vi "U3 Quadrature.vi"(8 "error in":errorcluster) -> (0 "error out":errorcluster)   [LabVIEW 2021]
panel:
  in  "Case Constant\n(See Context Help)":bool=TRUE
  in  "Stop":bool
  in  "Reset Count":bool
  out "Quadrature Count":i32
  in  "FirstFound":bool=TRUE
  in  "Address":string="1"
  out "Error Message":string
  # "Demonstrates 1 quadrature input, which uses two timer channels for phases A and B (FIO0 and FIO1 in this case).\nIf you don't have a quadrature signal source handy, you can connect wires to GND, and tap these wires on FIO0\nand FIO1 to simulate quadrature."
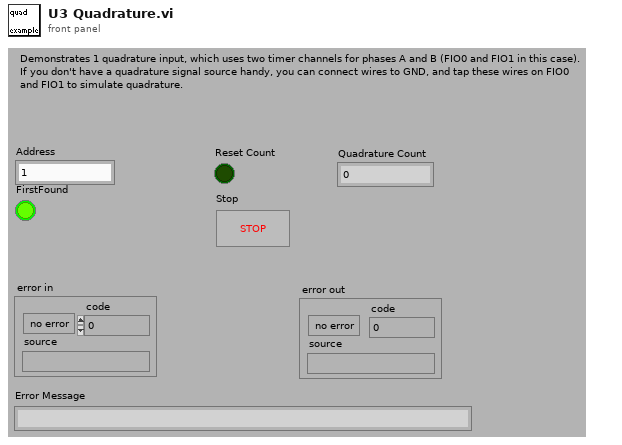
[diagram p1: front panel]
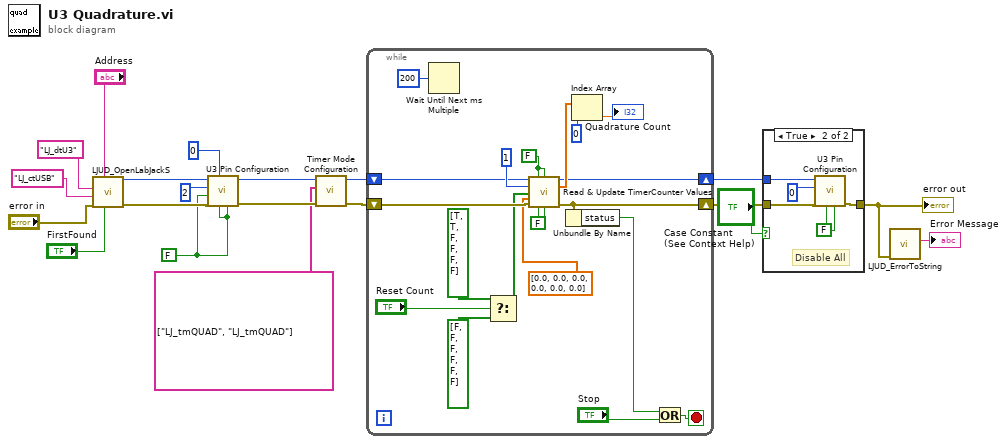
[diagram p0: block diagram]
diagram:
  w5 = FALSE ("Enable Counter0")
  n1 = call "LJUD_OpenLabJackS.vi"("FirstFound"="FirstFound", "Address"="Address", "error in"="error in", "ConnectionType"="LJ_ctUSB", "DeviceType"="LJ_dtU3") -> ("error out"=w8:errorcluster, "Handle"=w7:i32)  [unwired: 4 in, 1 out]
  n2 = call "U3 Pin Configuration.vi"("Enable Counter1"=w5, "Enable Counter0"=w5, "FIO/EIO Analog Enable"=0, "error in"=w8, "Enable DAC1"=w5, "Number of Timers Enabled"=2 ("# Timers Enabled"), "Handle In"=w7) -> ("error out"=w9:errorcluster, "Handle Out"=w6:i32)  [unwired: 3 in]
  n3 = call "Timer Mode Configuration.vi"("error in"=w9, "TimerModes"=string[] ["LJ_tmQUAD", "LJ_tmQUAD"], "Handle In"=w6) -> ("error out"=w14:errorcluster, "Handle Out"=w13:i32)  [unwired: 7 in]
  n4 = while {
    shift-right: [w32] -> w11
    shift-left: w13 -> [w34]
    shift-right: [w27] -> w12
    shift-left: w14 -> [w33]
    stop <- w26 stop-if-true
    w21 = FALSE ("Reset Counter0")
    w39 = FALSE ("Reset Counter0")
    n5 = Wait Until Next ms Multiple(millisecond multiple=u32 200) -> ()  [unwired: 1 out]
    n6 = Select(t=bool[] [TRUE, TRUE, FALSE, FALSE, FALSE, FALSE] ("UpdateReset Timers"), s="Reset Count", f=bool[] [FALSE, FALSE, FALSE, FALSE, FALSE, FALSE] ("UpdateReset Timers")) -> (s? t:f=w28:bool[])
    n7 = call "Read & Update TimerCounter Values.vi"("Handle In"=w34, "Reset Counter0"=w39, "Reset Counter1"=w39, "# Timers to Read"=1, "UpdateReset Timers"=w28, "TimerValues"=dbl[] [0.0, 0.0, 0.0, 0.0, 0.0, 0.0], "error in"=w33, "Read Counter0"=w21, "Read Counter1"=w21) -> ("Handle Out"=w32:i32, "Timer Value Reads"=w35:dbl[], "error out"=w27:errorcluster)  [unwired: 3 in, 1 out]
    n8 = Unbundle By Name(w27) -> ("status"=w25:bool)
    n9 = Index Array(array=w35, index=0 ("Index")) -> (element=→"Quadrature Count":dbl)
    n10 = Or(x=w25, y="Stop") -> (x .or. y?=w26:bool)
  }
  n11 = case shown="True" "Case Constant\n(See Context Help)" {
    tunnel: w12 -> [w40 w45]
    tunnel: w11 -> [_ w44]
    tunnel: [w40 w43] -> w16
    frame False {
    }
    frame True {
      w41 = FALSE ("Enable Counter0")
      # "Disable All"
      n12 = call "U3 Pin Configuration.vi"("Enable Counter1"=w41, "Enable Counter0"=w41, "error in"=w45, "Number of Timers Enabled"=0 ("# Timers Enabled"), "Handle In"=w44) -> ("error out"=w43:errorcluster)  [unwired: 5 in, 1 out]
    }
  }
  "error out" <- w16
  n13 = call "LJUD_ErrorToString.vi"("error in"=w16) -> ("String"=→"Error Message":string)  [unwired: 10 in]
